vi "Prompt for Step.vi"(8 "error in (no error)":errorcluster, 9 "Exit Event":refnum<user-event>, 10 "Subpanel Ref":refnum<vi>, 11 "Visible Assertion in":refnum<class "Visible Assertion.lvclass">) -> (0 "error out":errorcluster, 3 "Visible Assertion out":refnum<class "Visible Assertion.lvclass">)   [LabVIEW 2020, in "MacroAssert.lvlib" / "Visible Assertion.lvclass"]
uses:
  Visible Assertion.lvclass
  Visible Assertion.lvclass/Visible Assertion.ctl
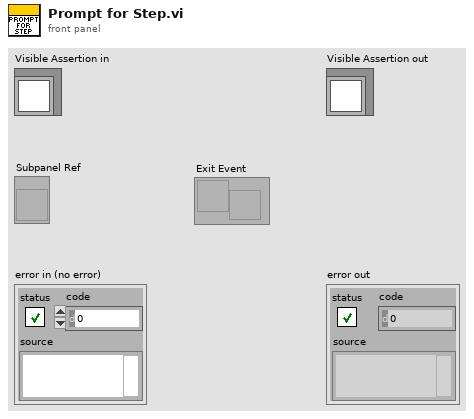
[diagram p1: front panel]
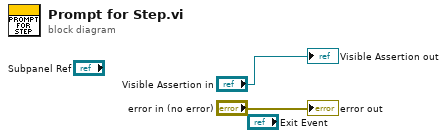
[diagram p0: block diagram]
diagram:
  "error out" <- "error in (no error)"
  "Visible Assertion out" <- "Visible Assertion in"
